vi "error_states.vi"(10 "mode":enum16{"read", "clear error", "set error"}(ring), 11 "error_code":T1) -> (3 "Error States":bool[](array[boolean]))   [LabVIEW 2011]
uses:
  error_codes.ctl
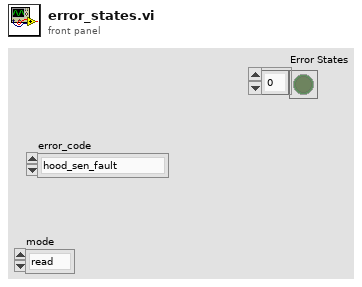
[diagram p1: front panel]
types:
  T1 = typedef "error_codes.ctl" = enum16{"hood_sen_fault", "turret_sen_fault", "peg_leg_sen_fault", "joe_johnson_sen_fault"}
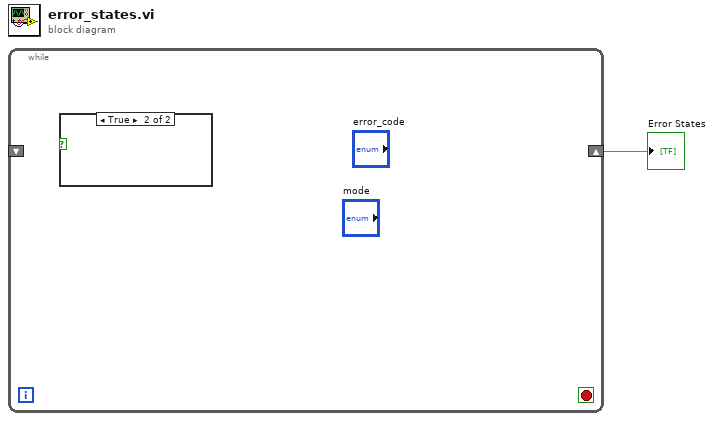
[diagram p0: block diagram]
diagram:
  n1 = while {
    shift-right: [_] -> w1
    shift-left: _ -> [_]
    stop <- _ stop-if-true
    n2 = case shown="True" {
      selector: _ -> [_ _]
      frame False {
      }
      frame True {
      }
    }
  }
  "Error States" <- w1
